vi "ExpEval_HandleOperator.vi"(9 "operator":string, 10 "expression in":string[](array[string]), 11 "Queue in":refnum<queue>) -> (1 "error":bool, 2 "expression out":string[](array[string]), 3 "Queue out":refnum<queue>)   [LabVIEW 2017, in "ExpressionEvaluator.lvlib"]
uses:
  <vilib>/addons/InsightCM/Utilities/ExpressionEvaluator/ExpressionEvaluator.lvlib
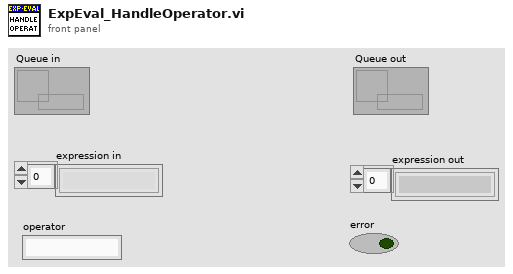
[diagram p1: front panel]
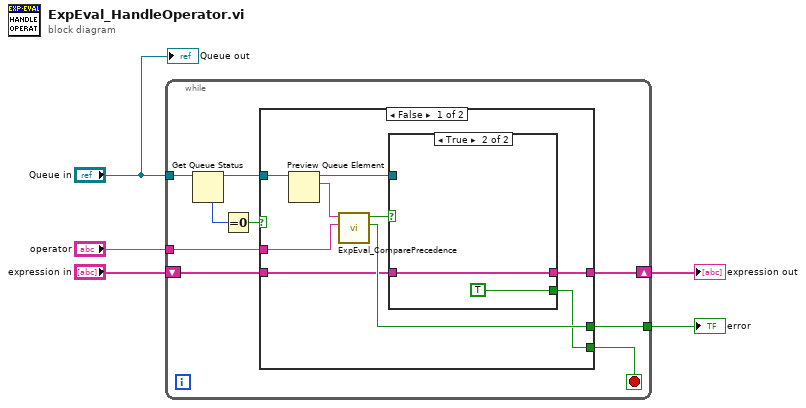
[diagram p0: block diagram]
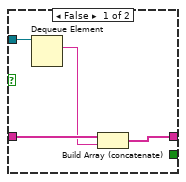
[diagram p2: hidden frame]
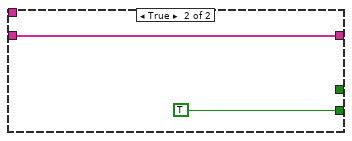
[diagram p3: hidden frame]
diagram:
  n1 = while {
    tunnel: "Queue in" -> [w14]
    tunnel: "operator" -> [w10]
    tunnel: [w9] -> w2
    shift-right: [w6] -> w5
    shift-left: "expression in" -> [w7]
    stop <- w8 stop-if-true
    n2 = Get Queue Status(queue=w14) -> (queue out=w11:refnum<queue>, # elements in queue=w13:i32)  [unwired: 2 in, 6 out]
    n3 = Equal To 0?(x=w13) -> (x = 0?=w12:bool)
    n4 = case shown="False" w12 {
      tunnel: w11 -> [w23 _]
      tunnel: w10 -> [w22 _]
      tunnel: [w19 _] -> w9
      tunnel: [w15 TRUE] -> w8
      tunnel: w7 -> [w17 w30]
      tunnel: [w16 w30] -> w6
      frame False {
        n5 = Preview Queue Element(queue=w23) -> (queue out=w18:refnum<queue>, element=w21:string)  [unwired: 2 in, 2 out]
        n6 = call <vilib>:"ExpEval_ComparePrecedence.vi"("Operator 2"=w22, "Operator 1"=w21) -> ("error"=w19:bool, "higher precedence"=w20:bool)  [unwired: 8 in]
        n7 = case shown="True" w20 {
          tunnel: w18 -> [w27 _]
          tunnel: w17 -> [w26 w29]
          tunnel: [w24 w29] -> w16
          tunnel: [_ TRUE] -> w15
          frame False {
            n8 = Dequeue Element(queue=w27) -> (element=w25:string)  [unwired: 2 in, 3 out]
            n9 = Build Array (concatenate)(w26, w25) -> (w24:string[])
          }
          frame True {
          }
        }
      }
      frame True {
      }
    }
  }
  "expression out" <- w5
  "error" <- w2
  "Queue out" <- "Queue in"
